vi "FdxCmdRxPortInitCvi.vi"(8 "error in":errorcluster, 9 "PortMap":u32, 11 "InstrumentHandle_port":u32) -> (0 "error out":errorcluster, 1 "PortInitOut":T1 {"PortConfig" items=["FDX_SINGLE", "FDX_REDUNDANT"]}, 3 "InstrumentHandle_port":u32)   [LabVIEW 2020, in "AIM664LV.lvlib"]
doc: "This function is for initializing the port. \nFor Receive functionality, the initialized state is as follows:\n- Global Statistics available\n- All Virtual Links, enabled for Activity information\n- Chronological Receive Mode, No VLs enabled for capturing\n- No Trigger Control Block Processing Enabled"
uses:
  AIM664LV.lvlib
  AFDX_LibraryAdmin/FdxGlobalDllPath.vi
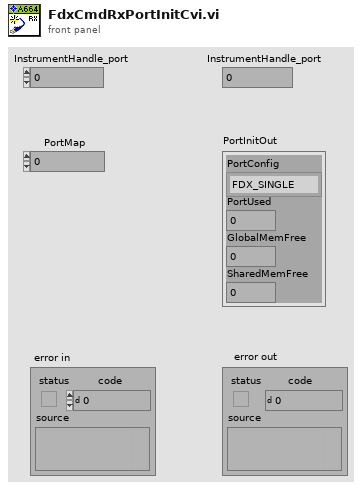
[diagram p1: front panel]
types:
  T1 = cluster{"PortConfig":u32, "PortUsed":u32, "GlobalMemFree":u32, "SharedMemFree":u32}
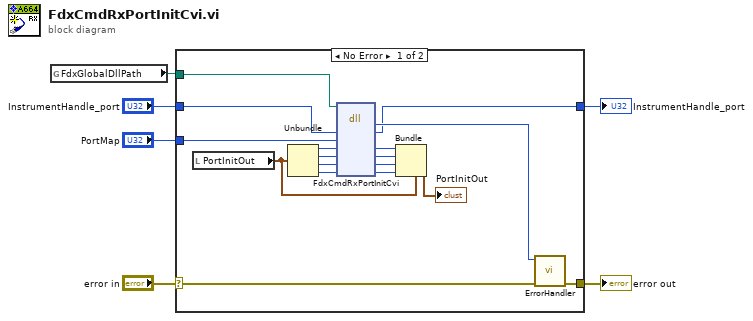
[diagram p0: block diagram]
diagram:
  n1 = global read "FdxGlobalDllPath.vi" "FdxGlobalDllPath"() -> (w4:path)
  n2 = case shown="No Error" "error in" {
    selector: "error in" -> [w22 w25]
    tunnel: [w23 w25] -> w6
    tunnel: w4 -> [w10 _]
    tunnel: [w9 w24] -> w3
    tunnel: "InstrumentHandle_port" -> [w8 w24]
    tunnel: "PortMap" -> [w7 _]
    frame No Error {
      n3 = local read "PortInitOut"() -> (w15:T1)
      n4 = Unbundle(w15) -> ("PortConfig"=w14:u32, "PortUsed"=w13:u32, "GlobalMemFree"=w12:u32, "SharedMemFree"=w11:u32)
      n5 = dll-call lib="aim_fdx.19.dll" fn="FdxCmdRxPortInitCvi"(path in=w10, "InstrumentHandle"=w8, "PortMap"=w7, "PortConfig"=w14, "PortUsed"=w13, "GlobalMemFree"=w12, "SharedMemFree"=w11) -> ("status"=w21:i32, "InstrumentHandle"=w9:u32, "PortConfig"=w19:u32, "PortUsed"=w18:u32, "GlobalMemFree"=w17:u32, "SharedMemFree"=w16:u32)  [unwired: 3 in, 2 out]
      n6 = Bundle(cluster=w15, "PortConfig"=w19, "PortUsed"=w18, "GlobalMemFree"=w17, "SharedMemFree"=w16) -> (→"PortInitOut":T1)
      n7 = call "ErrorHandler.vi"("error in"=w22, "AIM Error"=w21) -> ("error out"=w23:errorcluster)  [unwired: 9 in]
    }
    frame Error {
    }
  }
  "error out" <- w6
  "InstrumentHandle_port" <- w3
